vi "Obtain Mensaje from UI.vi"(8 "error in (no error)":errorcluster, 10 "Mensaje":string, 11 "Paquetes in":refnum<class "Paquetes.lvclass">) -> (0 "error out":errorcluster, 3 "Paquetes out":refnum<class "Paquetes.lvclass">)   [LabVIEW 2020, in "Paquetes.lvlib" / "Paquetes.lvclass"]
uses:
  Paquetes.lvclass
  Paquetes.lvclass/Paquetes.ctl
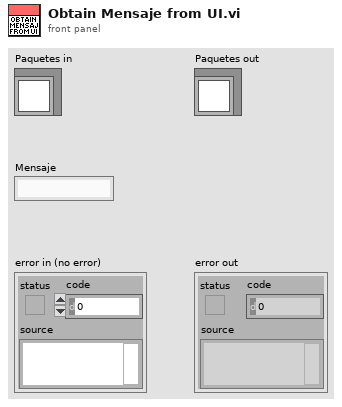
[diagram p1: front panel]
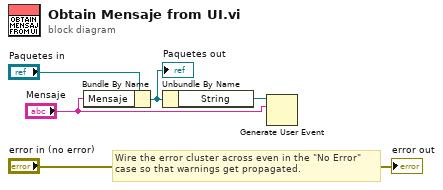
[diagram p0: block diagram]
diagram:
  # "Wire the error cluster across even in the \"No Error\"\ncase so that warnings get propagated."
  n1 = Bundle By Name(cluster="Paquetes in", "Mensaje"="Mensaje") -> (w3:refnum<class "Paquetes.lvclass">)
  "Paquetes out" <- w3
  n2 = Unbundle By Name(w3) -> ("String"=w2:refnum<user-event>)
  n3 = Generate User Event(user event=w2, event data cluster="Mensaje") -> ()  [unwired: 2 in, 2 out]
  "error out" <- "error in (no error)"
